vi "TOD Byte Stream to String.vi"(8 "error in (no error)":errorcluster, 10 "Byte Stream":u8[](array[numeric])) -> (0 "error out":errorcluster, 2 "Value":string)   [LabVIEW 2018, in "TwinCAT ADS.lvclass"]
uses:
  TwinCAT ADS.lvclass
  cb4a1201-b7c8-49b0-b8a9-7d7aff6d4c20.vi
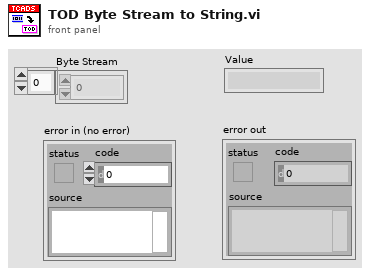
[diagram p1: front panel]
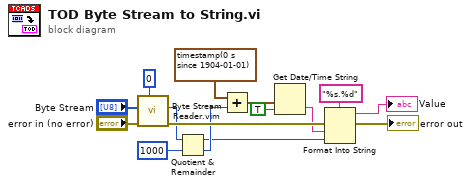
[diagram p0: block diagram]
diagram:
  n1 = call "Byte Stream Reader.vim"("Type"=u32 0, "error in (no error)"="error in (no error)", "Byte Stream"="Byte Stream") -> ("error out"=w15:errorcluster, "Value"=w7:u32)  [unwired: 7 in]
  n2 = Quotient & Remainder(x=w7, y=u32 1000) -> (x-y*floor(x/y)=w6:u32, floor(x/y)=w11:u32)
  n3 = Add(x=timestamp(0 s since 1904-01-01), y=w11) -> (x+y=w10:timestamp)
  n4 = Get Date/Time String(seconds (now)=w10, want seconds? (F)=TRUE) -> (time string=w5:string)  [unwired: 1 in, 1 out]
  n5 = Format Into String(format string="%s.%d", error in=w15, w5, w6) -> (resulting string=→"Value":string, error out=→"error out":errorcluster)  [unwired: 1 in]
